vi "sendValue.vi"(8 "error in (no error)":errorcluster, 10 "data":variant, 11 "Timestamp in":refnum<class "timestamp.lvclass">) -> (0 "error out":errorcluster, 2 "function return":i32, 3 "Timestamp out":refnum<class "timestamp.lvclass">)   [LabVIEW 2016, in "SALLV_AtDome_Messaging.lvlib" / "timestamp.lvclass"]
uses:
  timestamp.lvclass
  ts_sallv_AtDome/DataTypes/timestamp.ctl
  timestamp.lvclass/timestamp.ctl
  ts_sallv_AtDome/SALLV_AtDome.lvlib
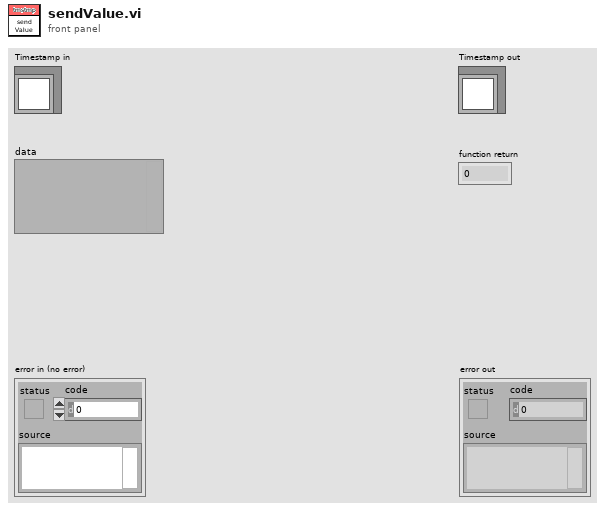
[diagram p1: front panel]
types:
  T1 = typedef "SALLV_AtDome.lvlib/timestamp.ctl" = cluster{"timestamp":dbl}
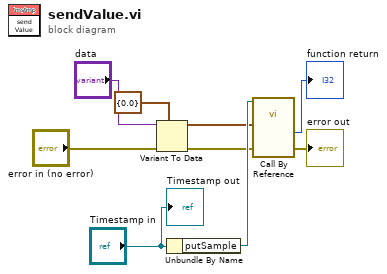
[diagram p0: block diagram]
diagram:
  n1 = Variant To Data(error in="error in (no error)", type=T1 {"timestamp"=0.0} ("timestamp_Ctl"), Variant="data") -> (data=w4:T1, error out=w3:errorcluster)
  n2 = Unbundle By Name("Timestamp in") -> ("putSample"=w6:refnum<vi>)
  n3 = call-by-ref "?"(reference=w6, "error in (no error)"=w3, "timestamp_Ctl"=w4) -> ("error out"=→"error out":errorcluster, "function return"=→"function return":i32)  [unwired: 8 in, 3 out]
  "Timestamp out" <- "Timestamp in"
